vi "Arrow_Globals.vi"() -> ()   [LabVIEW 2020]
uses:
  Subsystems/Arrow/Arrow_Cluster.ctl
  Subsystems/Arrow/Arrow_Control_States.ctl
panel:
  in  "Arrow_Motor_Output":dbl
  in  "Arrow_Execute_Notifier":refnum<notifier>
  in  "Arrow_Set_Notifier":refnum<notifier>
  in  "Arrow_Execute_Ref":string="Arrow_Execute_Ref"
  in  "Arrow_Set_Ref":string="Arrow_Set_Ref"
  in  "Arrow_Motor":string="Arrow_Motor"
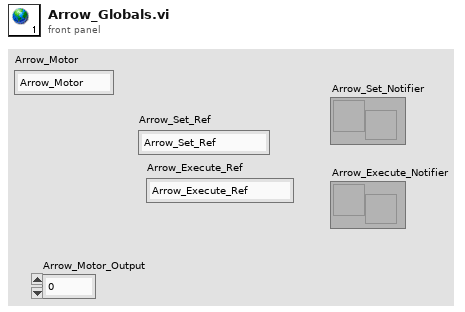
[diagram p1: front panel]
diagram:
